vi "Read To Char.vi"(6 "Char":string, 8 "error in (no error)":errorcluster, 11 "VisaComms in":refnum<class "VisaComms.lvclass">) -> (0 "error out":errorcluster, 2 "Response":string, 3 "VisaComms out":refnum<class "VisaComms.lvclass">)   [LabVIEW 2024, in "CTI.lvlib" / "VisaComms.lvclass"]
uses:
  VisaComms.lvclass
  VisaComms.lvclass/VisaComms.ctl
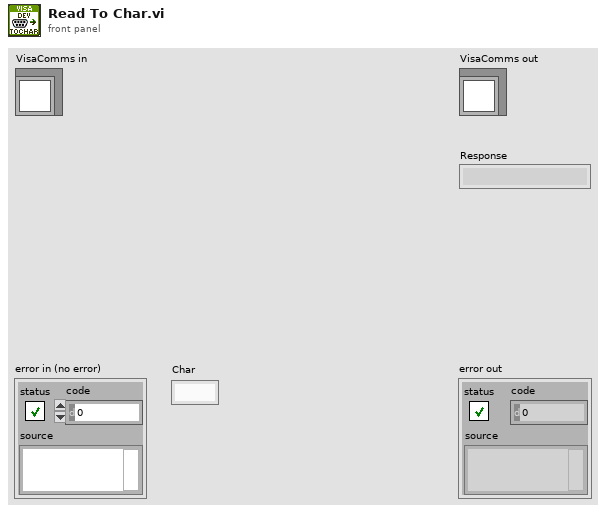
[diagram p1: front panel]
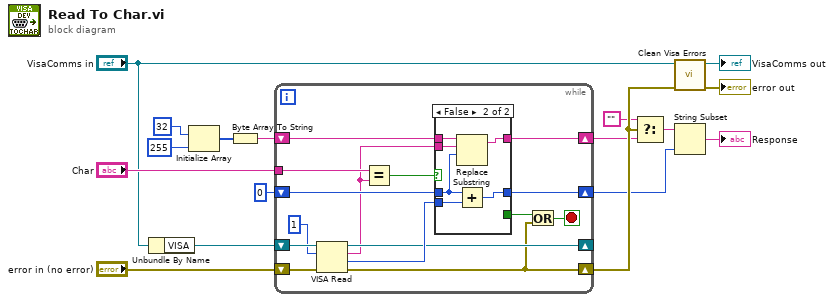
[diagram p0: block diagram]
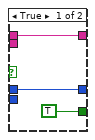
[diagram p2: hidden frame]
diagram:
  n1 = Unbundle By Name("VisaComms in") -> ("VISA"=w5:refnum<visa-resource-name>)
  n2 = Initialize Array(u8 32 ("element"), 255 ("dimension size")) -> (w3:u8[])
  n3 = Byte Array To String(unsigned byte array=w3) -> (string=w14:string)
  n4 = while {
    shift-right: [w22] -> w17
    shift-left: "error in (no error)" -> [w31]
    shift-right: [w23] -> _
    shift-left: w5 -> [w32]
    shift-right: [w26] -> w13
    shift-left: w14 -> [w29]
    shift-right: [w27] -> w10
    shift-left: u32 0 -> [w28]
    tunnel: "Char" -> [w20]
    stop <- w24 stop-if-true
    n5 = VISA Read(VISA resource name=w32, byte count=u32 1, error in (no error)=w31) -> (VISA resource name out=w23:refnum<visa-resource-name>, read buffer=w18:string, return count=w25:u32, error out=w22:errorcluster)
    n6 = Equal?(x=w20, y=w18) -> (x = y?=w19:bool)
    n7 = case shown="False" w19 {
      tunnel: w29 -> [w35 w41]
      tunnel: w28 -> [w34 w40]
      tunnel: [w34 w39] -> w27
      tunnel: [w35 w38] -> w26
      tunnel: w25 -> [_ w37]
      tunnel: [TRUE _] -> w21
      tunnel: w18 -> [_ w36]
      frame True {
      }
      frame False {
        n8 = Replace Substring(3:w40, 4:w36, 5:w41) -> (1:w38:string)  [unwired: 1 in, 1 out]
        n9 = Add(x=w40, y=w37) -> (x+y=w39:u32)
      }
    }
    n10 = Or(x=w21, y=w22) -> (x .or. y?=w24:bool)
  }
  n11 = Select(t="", s=w17, f=w13) -> (s? t:f=w11:string)
  n12 = call "Clean Visa Errors.vi"("error in (no error)"=w17, "VisaComms in"="VisaComms in") -> ("error out"=→"error out":errorcluster, "VisaComms out"=→"VisaComms out":refnum<class "VisaComms.lvclass">)  [unwired: 8 in]
  n13 = String Subset(string=w11, length (rest)=w10) -> (substring=→"Response":string)  [unwired: 1 in]
